vi "One angle test.vi"() -> ()   [LabVIEW 2010]
uses:
  ROS/Code/SubVIs/JointMode.ctl
  ROS/Code/SubVIs/BaxterArmsSmall.ctl
  ROS/Code/SubVIs/BaxterSide.ctl
panel:
  out "T sample":dbl
  in  "Elbow 0 desired angle":dbl=45.0
  in  "Gain":dbl=4.0
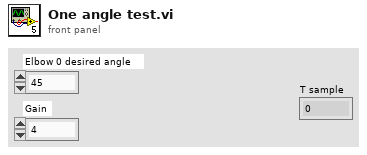
[diagram p1: front panel]
types:
  T1 = typedef "BaxterArmsSmall.ctl" = cluster{"Elbow 0":dbl, "Elbow 1":dbl, "Shoulder 0":dbl, "Shoulder 1":dbl, "Wrist 0":dbl, "Wrist 1":dbl, "Wrist 2":dbl}
  T2 = typedef "BaxterSide.ctl" = enum16{"left", "right"}
  T3 = enum16{"left_e0", "left_e1", "left_s0", "left_s1", "left_w0", "left_w1", "left_w2", "right_e0", "right_e1", "right_s0", "right_s1", "right_w0", "right_w1", "right_w2"}
  T4 = typedef "JointMode.ctl" = u8
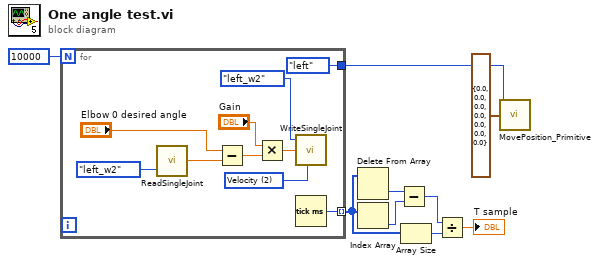
[diagram p0: block diagram]
diagram:
  n1 = for {
    N: 10000 -> [_]
    tunnel: [w19] -> w5 mode=indexing
    tunnel: [BaxterSide."left" ("Side")] -> w1
    w14 = T4 2 items=["Position"=1, "Velocity"=2, "Effort"=3] ("Mode")
    n2 = call "ReadSingleJoint.vi"("Angle Name"=T3."left_w2") -> ("Position"=w12:dbl)  [unwired: 1 in, 2 out]
    n3 = Subtract(x="Elbow 0 desired angle", y=w12) -> (x-y=w18:dbl)
    n4 = Multiply(x="Gain", y=w18) -> (x*y=w16:dbl)
    n5 = call "WriteSingleJoint.vi"("Angle Name"=T3."left_w2", "Angle (degrees)"=w16, "Mode"=w14) -> ()  [unwired: 3 in, 1 out]
    n6 = Tick Count (ms)() -> (millisecond timer value=w19:u32)
  }
  n7 = Delete From Array(array=w5) -> (deleted portion=w8:u32)  [unwired: 2 in, 1 out]
  n8 = Index Array(array=w5) -> (element=w7:u32)  [unwired: 1 in]
  n9 = Subtract(x=w8, y=w7) -> (x-y=w6:u32)
  n10 = Array Size(array=w5) -> (size(s)=w4:i32)
  n11 = Divide(x=w6, y=w4) -> (x/y=→"T sample":dbl)
  n12 = call "MovePosition_Primitive.vi"("Side"=w1, "Arm Angles (degrees)"=T1 {"Elbow 0"=0.0, "Elbow 1"=0.0, "Shoulder 0"=0.0, "Shoulder 1"=0.0, "Wrist 0"=0.0, "Wrist 1"=0.0, "Wrist 2"=0.0}) -> ()  [unwired: 4 in, 1 out]
